vi "Tab_controls_color_example.vi"() -> ()   [LabVIEW 2018]
panel:
  in  "Registerkarte":enum32{"Seite 1", "Seite 2"}(tab)
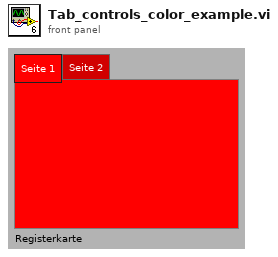
[diagram p1: front panel]
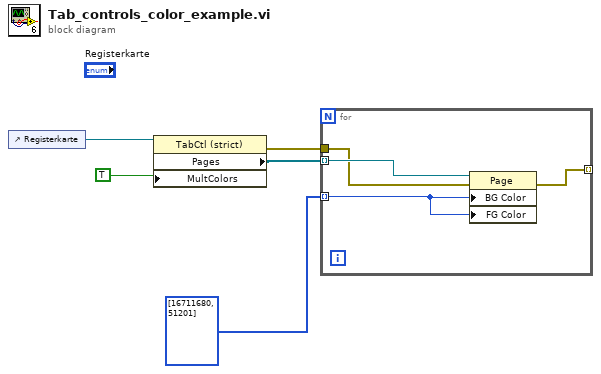
[diagram p0: block diagram]
diagram:
  n1 = control-ref of="Registerkarte"() -> (w5:refnum<vi>)
  n2 = property class="TabCtl (strict)"(reference=w5, "MultColors"=TRUE ("Mehrere Farben zulassen")) -> (error out=w2:errorcluster, "Pages"=w4:refnum<vi>[])  [unwired: 1 in, 1 out]
  n3 = for {
    tunnel: w4 -> [w9] mode=indexing
    tunnel: u32[] [16711680, 51201] -> [w8] mode=indexing
    tunnel: w2 -> [w7]
    tunnel: [w6] -> _ mode=indexing
    n4 = property class="Page"(reference=w9, error in=w7, "BG Color"=w8, "FG Color"=w8) -> (error out=w6:errorcluster)  [unwired: 1 out]
  }
